vi "Step_1_Ans_PS.vi"   [LabVIEW 2012]
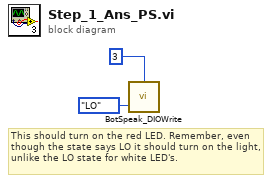
[diagram p0: block diagram]
diagram:
  # "This should turn on the red LED. Remember, even though the state says LO it should turn on the light, unlike the LO state for white LED's."
  n1 = call <userlib>:"BotSpeak_DIOWrite.vi"("State"=enum32{"LO", "HI"}."LO", "DIO Line"=u32 3) -> ()  [unwired: 1 in, 2 out]
